vi "Read Ethernet Config.vi"() -> (0 "error out":errorcluster)   [LabVIEW 2020]
panel:
  out "Values (other)":dbl[](array[numeric]) format="%.2f"
  in  "Names (other)":string[](array[string])=["ETHERNET_DHCP_ENABLE", "ETHERNET_DHCP_ENABLE_DEFAULT"]
  out "NumberToIP":string[](array[string])
  out "Error String":string
  out "ConnectionType Out":i32
  out "DeviceType Out":i32
  in  "Identifier":string="LJM_idANY"
  in  "ConnectionType":string="LJM_ctANY"
  in  "DeviceType":string="LJM_dtANY"
  out "Values (IP)":dbl[](array[numeric]) format="%.2f"
  in  "Names (IP)":string[](array[string])=["ETHERNET_IP", "ETHERNET_SUBNET", "ETHERNET_GATEWAY", "ETHERNET_IP_DEFAULT", "ETHERNET_SUBNET_DEFAULT", "ETHERNET_GATEWAY_DEFAULT"]
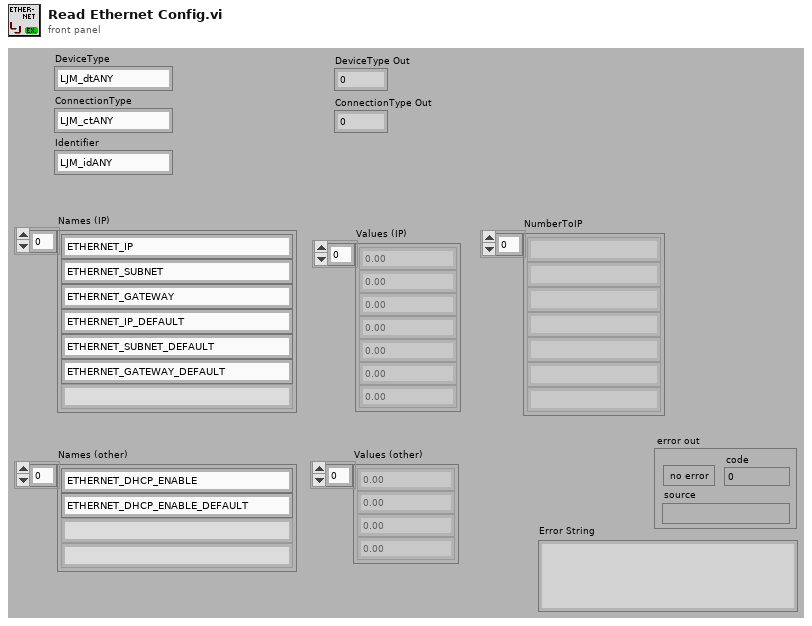
[diagram p1: front panel]
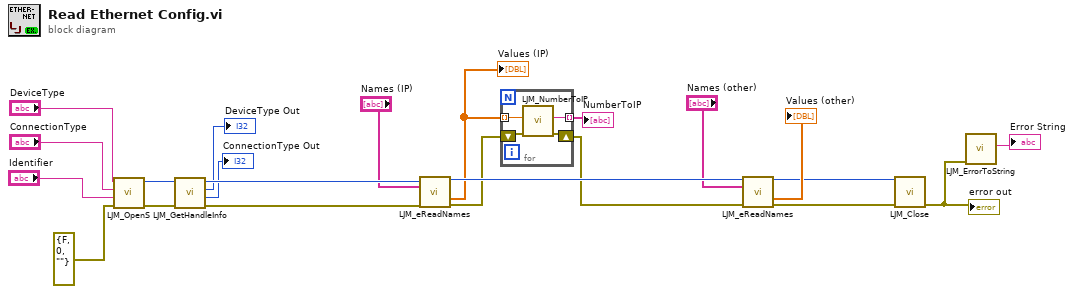
[diagram p0: block diagram]
diagram:
  n1 = call "LJM_OpenS.vi"("error in"=errorcluster {"status"=FALSE, "code"=0, "source"=""} ("error in (no error)"), "Identifier"="Identifier", "ConnectionType"="ConnectionType", "DeviceType"="DeviceType") -> ("error out"=w21:errorcluster, "Handle"=w19:i32)  [unwired: 6 in]
  n2 = call "LJM_GetHandleInfo.vi"("error in"=w21, "Handle In"=w19) -> ("error out"=w20:errorcluster, "ConnectionType"=→"ConnectionType Out":i32, "DeviceType"=→"DeviceType Out":i32, "Handle Out"=w18:i32)  [unwired: 2 in, 4 out]
  n3 = call "LJM_eReadNames.vi"("Handle In"=w18, "aNames"="Names (IP)", "error in"=w20) -> ("Handle Out"=w9:i32, "aValuesOut"=w6:dbl[], "error out"=w2:errorcluster)  [unwired: 9 in, 1 out]
  "Values (IP)" <- w6
  n4 = for {
    tunnel: w6 -> [w26] mode=indexing
    tunnel: [w25] -> w5 mode=indexing
    shift-right: [w23] -> w1
    shift-left: w2 -> [w24]
    n5 = call "LJM_NumberToIP.vi"("error in"=w24, "Number"=w26) -> ("error out"=w23:errorcluster, "IPv4String"=w25:string)  [unwired: 8 in]
  }
  "NumberToIP" <- w5
  n6 = call "LJM_eReadNames.vi"("Handle In"=w9, "aNames"="Names (other)", "error in"=w1) -> ("Handle Out"=w4:i32, "aValuesOut"=→"Values (other)":dbl[], "error out"=w3:errorcluster)  [unwired: 9 in, 1 out]
  n7 = call "LJM_Close.vi"("error in"=w3, "Handle"=w4) -> ("error out"=w12:errorcluster)  [unwired: 9 in]
  "error out" <- w12
  n8 = call "LJM_ErrorToString.vi"("error in"=w12) -> ("String"=→"Error String":string)  [unwired: 10 in]
